vi "ChannelSelectionScreen.vi"(8 "error in":errorcluster, 10 "Selected Channels":T1 {"Input Channels"."Node Ref" format="%.0x"}, 11 "Parent Ref":T3=18446744073709551615 format="%.0x") -> (0 "error out":errorcluster, 1 "Cancelled?":bool, 2 "Selected Channels":T1 {"Input Channels"."Node Ref" format="%.0x"}, 3 "Parent Ref Out":T3=18446744073709551615 format="%.0x")   [LabVIEW 2015, in "J1939 Addon System Explorer.lvlib"]
uses:
  J1939 Addon System Explorer.lvlib
  NationalInstruments.VeriStand.SystemStorageUI
  <vilib>/NI Veristand/Custom Device API/Custom Device Item Ref.ctl
  Types/Protection Signal Settings.ctl
  Types/Protection Signal Linked Channels.ctl
  Shared/Types/Protection Type.ctl
  <vilib>/NI VeriStand/Custom Device API/Custom Device API.lvlib
  Shared/J1939 Addon Shared.lvlib
panel:
  in  "Cancel":bool
  in  "OK":bool
  in  "Protection Data":refnum<k24>(container)
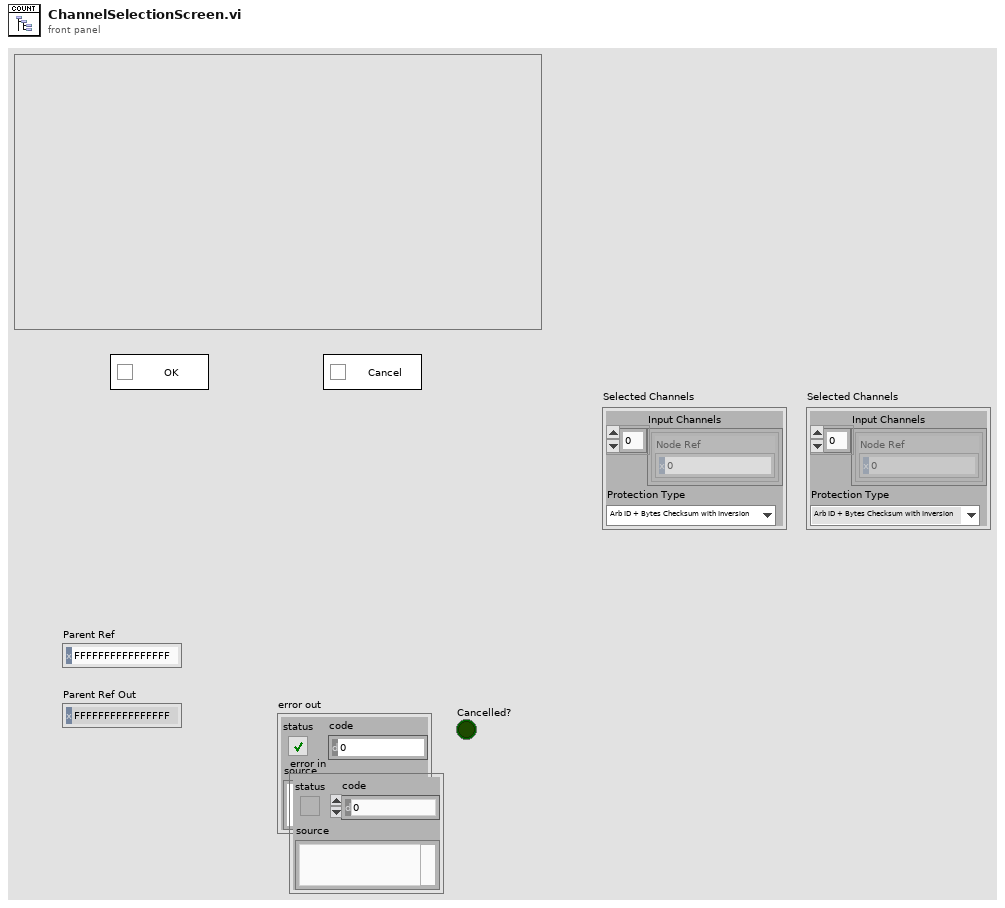
[diagram p1: front panel]
types:
  T1 = typedef "J1939 Addon System Explorer.lvlib/Protection Signal Settings.ctl" = cluster{"Input Channels":T2[], "Protection Type":T4}
  T2 = typedef "J1939 Addon System Explorer.lvlib/Protection Signal Linked Channels.ctl" = cluster{"Node Ref":T3}
  T3 = typedef "Custom Device API.lvlib/Custom Device Item Ref.ctl" = u64
  T4 = typedef "J1939 Addon Shared.lvlib/Protection Type.ctl" = enum16{"Arb ID + Bytes Checksum with Inversion", "Arb ID + Bytes CRC with Inversion", "Reversed Raw Signal Checksum with Inversion"}
  T5 = typedef "Custom Device API.lvlib/Custom Device Pointer.ctl" = refnum<k24>
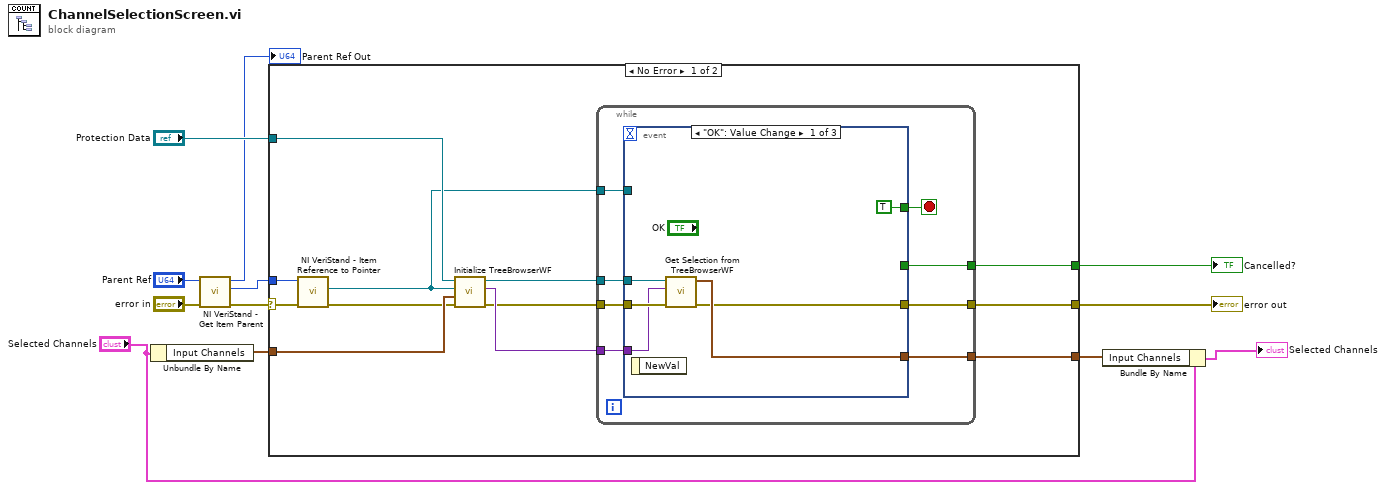
[diagram p0: block diagram]
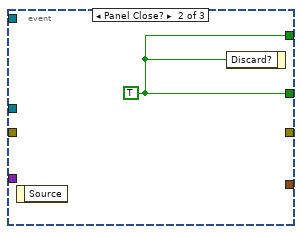
[diagram p2: hidden frame]
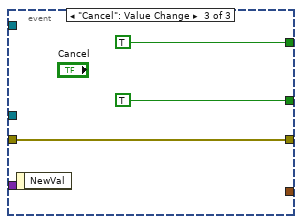
[diagram p3: hidden frame]
diagram:
  n1 = Unbundle By Name("Selected Channels") -> ("Input Channels"=w9:T2[])
  n2 = call <vilib>:"NI VeriStand - Get Item Parent.vi"("error in (no error)"="error in", "Item Ref in"="Parent Ref") -> ("error out"=w3:errorcluster, "Parent Ref"=w1:T3, "Item Ref out"=→"Parent Ref Out":T3)  [unwired: 6 in, 1 out]
  n3 = case shown="No Error" w3 {
    selector: w3 -> [w23 w43]
    tunnel: "Protection Data" -> [w19 _]
    tunnel: w1 -> [w24 _]
    tunnel: [w22 _] -> w11
    tunnel: [w16 w43] -> w10
    tunnel: [w21 _] -> w8
    tunnel: w9 -> [w20 _]
    frame No Error {
      n4 = call <vilib>:"NI VeriStand - Item Reference to Pointer.vi"("error in (no error)"=w23, "Item Ref in"=w24) -> ("error out"=w15:errorcluster, "Node Pointer"=w14:T5)  [unwired: 6 in, 2 out]
      n5 = call "Initialize TreeBrowserWF.vi"("error in (no error)"=w15, "Input Channels"=w20, "Node Pointer"=w14, "TreeBrowserRef"=w19) -> ("error out"=w13:errorcluster, "Channels"=w18:variant, "TreeBrowserRef 2"=w17:refnum<k24>)  [unwired: 5 in]
      n6 = while {
        tunnel: w13 -> [w32]
        tunnel: w17 -> [w31]
        tunnel: [w29] -> w22
        tunnel: [w28] -> w16
        tunnel: [w27] -> w21
        tunnel: w18 -> [w26]
        tunnel: w14 -> [w25]
        stop <- w30 stop-if-true
        n7 = event shown="[0] \"OK\": Value Change" {
          selector: _ -> [_ _ _]
          dyn-events: _ -> [_ _ _]
          timeout: _ -> [_ _ _]
          tunnel: w32 -> [w38 _ w42]
          tunnel: w31 -> [w37 _ _]
          tunnel: [w34 _ w42] -> w28
          tunnel: [TRUE w39 TRUE] -> w30
          tunnel: [_ w39 TRUE] -> w29
          tunnel: [w35 _ _] -> w27
          tunnel: w26 -> [w36 _ _]
          tunnel: w25 -> [_ _ _]
          event "OK": Value Change {
            n8 = event-data() -> ()  [unwired: 1 in, 1 out]
            n9 = call "Get Selection from TreeBrowserWF.vi"("error in (no error)"=w38, "Input Channels"=w36, ".NET Refnum in"=w37) -> ("error out"=w34:errorcluster, "Input Channel Selections"=w35:T2[])  [unwired: 7 in]
          }
          event Panel Close? {
            w39 = TRUE
            n10 = event-data() -> ()  [unwired: 1 in, 1 out]
            n11 = event-data("Discard?"=w39) -> ()  [unwired: 1 in, 1 out]
          }
          event "Cancel": Value Change {
            n12 = event-data() -> ()  [unwired: 1 in, 1 out]
          }
        }
      }
    }
    frame Error {
    }
  }
  "Cancelled?" <- w11
  "error out" <- w10
  n13 = Bundle By Name(cluster="Selected Channels", "Input Channels"=w8) -> (→"Selected Channels":T1)
